vi "DBToString.vi"(1 "Enum":T1) -> (0 "Refname":string)   [LabVIEW 2013]
uses:
  DBNameEnum.ctl
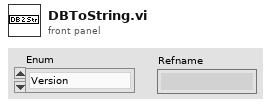
[diagram p1: front panel]
types:
  T1 = typedef "DBNameEnum.ctl" = enum16{"Version"}
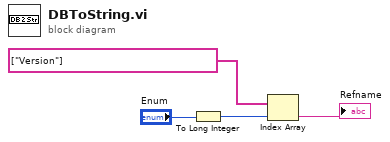
[diagram p0: block diagram]
diagram:
  n1 = To Long Integer(number="Enum") -> (32bit integer=w1:i32)
  n2 = Index Array(array=string[] ["Version"] ("RefnameArray"), index=w1) -> (element=→"Refname":string)
